vi "getFGenDevices.vi"() -> (0 "Array":T1(array[cluster]))   [LabVIEW 2015]
uses:
  <instrlib>/niModInst/niModInst Get Installed Device Attribute (String).vi
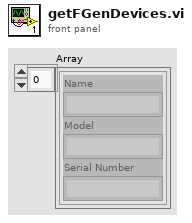
[diagram p1: front panel]
types:
  T1 = cluster{"Name":string, "Model":string, "Serial Number":string}[]
  T2 = cluster{"Name":string, "Model":string, "Serial Number":string}
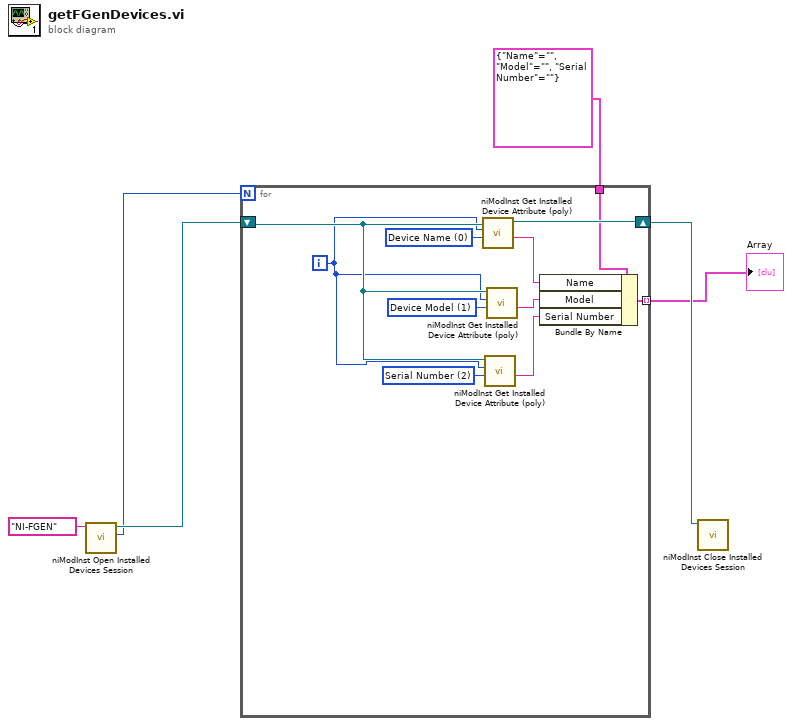
[diagram p0: block diagram]
diagram:
  n1 = call <instrlib>:"niModInst Open Installed Devices Session.vi"("driver"="NI-FGEN") -> ("device count"=w4:i32, "session"=w5:refnum<k20>)  [unwired: 8 in, 1 out]
  n2 = for {
    N: w4 -> [_]
    shift-right: [w17] -> w3
    shift-left: w5 -> [w13]
    tunnel: T2 {"Name"="", "Model"="", "Serial Number"=""} -> [w12]
    tunnel: [w11] -> w1 mode=indexing
    i -> [w7]
    w14 = 2 items=["Device Name", "Device Model", "Serial Number"] ("attribute ID")
    w15 = 1 items=["Device Name", "Device Model", "Serial Number"] ("attribute ID")
    w16 = 0 items=["Device Name", "Device Model", "Serial Number"] ("attribute ID")
    n3 = call-poly <instrlib>:"niModInst Get Installed Device Attribute (poly).vi"("attribute ID"=w16, "index in"=w7, "session in"=w13) -> ("attribute value"=w10:string, "session out"=w17:refnum<k20>)  [unwired: 5 in, 2 out]
    n4 = call-poly <instrlib>:"niModInst Get Installed Device Attribute (poly).vi"("attribute ID"=w14, "index in"=w7, "session in"=w13) -> ("attribute value"=w8:string)  [unwired: 5 in, 3 out]
    n5 = call-poly <instrlib>:"niModInst Get Installed Device Attribute (poly).vi"("attribute ID"=w15, "index in"=w7, "session in"=w13) -> ("attribute value"=w9:string)  [unwired: 5 in, 3 out]
    n6 = Bundle By Name(cluster=w12, "Name"=w10, "Model"=w9, "Serial Number"=w8) -> (w11:T2)
  }
  "Array" <- w1
  n7 = call <instrlib>:"niModInst Close Installed Devices Session.vi"("session"=w3) -> ()  [unwired: 10 in, 1 out]
